vi "Get Service Descriptor.vi"(8 "error in":errorcluster, 11 "Continuous Counting Mesurement2 in":refnum<class "Continuous Counting Measurement2.lvclass">) -> (0 "error out":errorcluster, 2 "service descriptor":T1, 3 "Continuous Counting Mesurement2 out":refnum<class "Continuous Counting Measurement2.lvclass">)   [LabVIEW 2021, in "MeasurementServerTests.lvlib" / "Measurement Service Tests.lvlib" / "Continuous Counting Measurement2.lvclass"]
doc: "Provides metadata used to describe and identify the measurement."
uses:
  Continuous Counting Measurement2.lvclass
  Runtime/Measurements/Helpers/TypeDefs/Service Descriptor.ctl
  Runtime/Measurements/Helpers/TypeDefs/Measurement Details.ctl
  Runtime/Measurements/Helpers/TypeDefs/Measurement Annotation.ctl
  Runtime/Measurements/NI Measurement Plug-In SDK.lvlib
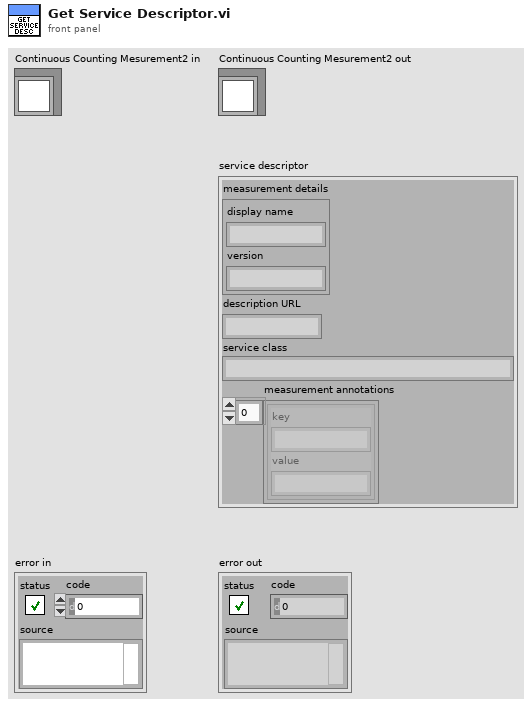
[diagram p1: front panel]
types:
  T1 = typedef "NI Measurement Plug-In SDK.lvlib/Service Descriptor.ctl" = cluster{"measurement details":T2, "description URL":string, "service class":string, "measurement annotations":T3[]}
  T2 = typedef "NI Measurement Plug-In SDK.lvlib/Measurement Details.ctl" = cluster{"display name":string, "version":string}
  T3 = typedef "NI Measurement Plug-In SDK.lvlib/Measurement Annotation.ctl" = cluster{"key":string, "value":string}
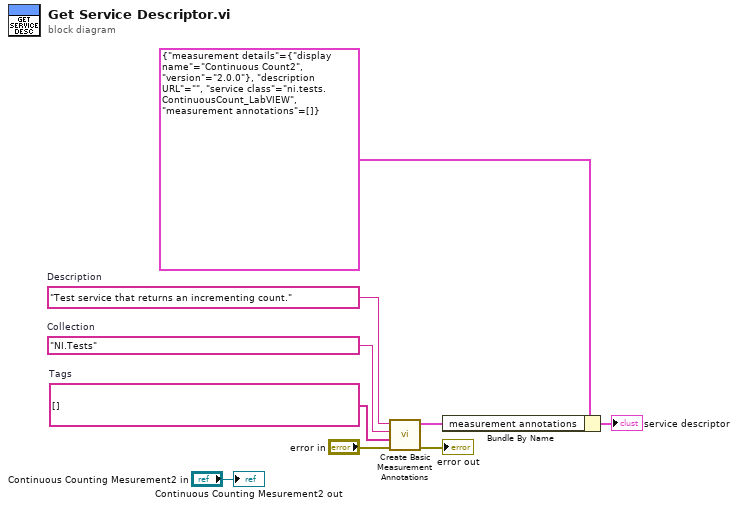
[diagram p0: block diagram]
diagram:
  w6 = string[] []  # Tags
  w7 = "NI.Tests"  # Collection
  w8 = "Test service that returns an incrementing count."  # Description
  n1 = call "Create Basic Measurement Annotations.vi"("error in"="error in", "tags"=w6, "collection"=w7, "description"=w8) -> ("error out"=→"error out":errorcluster, "measurement annotations"=w2:T3[])  [unwired: 6 in]
  n2 = Bundle By Name(cluster=T1 {"measurement details"={"display name"="Continuous Count2", "version"="2.0.0"}, "description URL"="", "service class"="ni.tests.ContinuousCount_LabVIEW", "measurement annotations"=[]} ("service descriptor"), "measurement annotations"=w2) -> (→"service descriptor":T1)
  "Continuous Counting Mesurement2 out" <- "Continuous Counting Mesurement2 in"
